vi "Example Threshold - Humidity Callback.vi"(4 "HumidityReached":refnum<user-event>, 5 "Event Data":cluster{"sender":refnum<k24>, "humidity":i32}, 6 "Control Ref":refnum<k24>, 7 "Event Common Data":T1) -> ()   [LabVIEW 2010]
uses:
  C:/tf/play/labview/Tinkerforge.dll
  Tinkerforge.dll
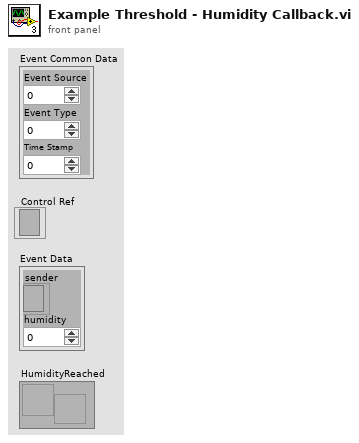
[diagram p1: front panel]
types:
  T1 = cluster{"Event Source":i32, "Event Type":u32, "Time Stamp":u32}
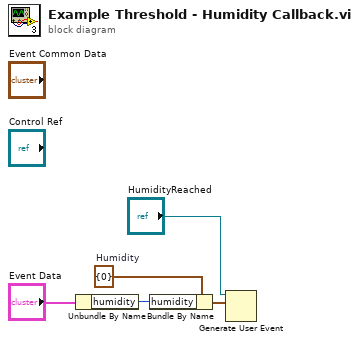
[diagram p0: block diagram]
diagram:
  w4 = cluster{"humidity":i32} {"humidity"=0}  # Humidity
  n1 = Unbundle By Name("Event Data") -> ("humidity"=w3:i32)
  n2 = Bundle By Name(cluster=w4, "humidity"=w3) -> (w1:cluster{"humidity":i32})
  n3 = Generate User Event(user event="HumidityReached", event data cluster=w1) -> ()  [unwired: 1 in, 2 out]
